vi "Binomial CDF.vi"(9 "p":dbl=0.02, 10 "n":i32=100, 11 "x":dbl) -> (0 "error":i32, 3 "cdf(x)":dbl=0.13261955589475294)   [LabVIEW 2020, in "NI_Gmath.lvlib"]
doc: "Computes the discrete cumulative distribution function (CDF), or the probability that the random variate X, where X describes the selected distribution type, takes on a value less than or equal to <B>x</B>. You must manually select the polymorphic instance to use."
uses:
  <vilib>/gmath/NI_Gmath.lvlib
  <vilib>/gmath/statdist.llb/st_error_code.ctl
  <vilib>/gmath/SpecialFunctions.llb/Incomplete Beta Function.vi
panel:
  # "Binomial CDF"
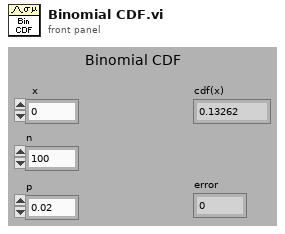
[diagram p1: front panel]
types:
  T1 = typedef "NI_Gmath.lvlib/st_error_code.ctl" = i32
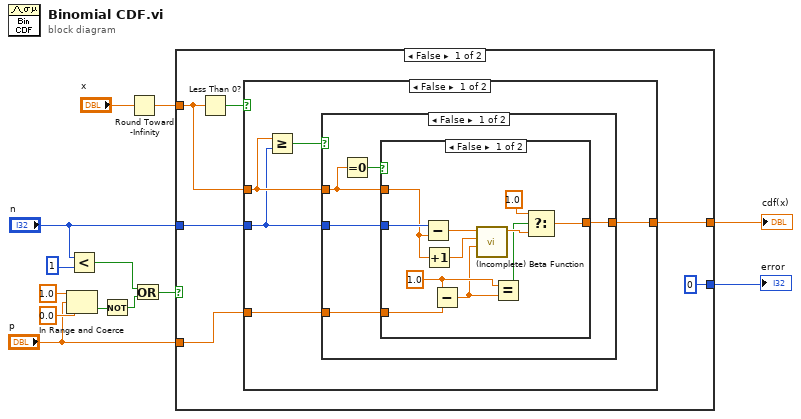
[diagram p0: block diagram]
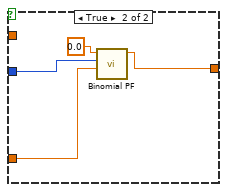
[diagram p2: hidden frame]
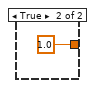
[diagram p3: hidden frame]
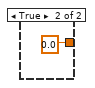
[diagram p4: hidden frame]
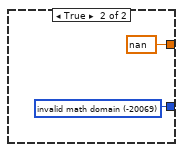
[diagram p5: hidden frame]
diagram:
  n1 = In Range and Coerce(upper limit=1.0, x="p", lower limit=0.0) -> (In Range?=w5:bool)  [unwired: 1 out]
  n2 = Less?(x="n", y=1) -> (x < y?=w3:bool)
  n3 = Not(x=w5) -> (.not. x?=w4:bool)
  n4 = Round Toward -Infinity(1:"x") -> (0:w1:dbl)
  n5 = Or(x=w3, y=w4) -> (x .or. y?=w8:bool)
  n6 = case shown="False" w8 {
    tunnel: [0 ("invalid math domain") w47] -> w13
    tunnel: [w18 nan] -> w12
    tunnel: w1 -> [w14 _]
    tunnel: "n" -> [w17 _]
    tunnel: "p" -> [w16 _]
    frame False {
      n7 = Less Than 0?(x=w14) -> (x < 0?=w15:bool)
      n8 = case shown="False" w15 {
        tunnel: [w23 0.0] -> w18
        tunnel: w14 -> [w22 _]
        tunnel: w17 -> [w21 _]
        tunnel: w16 -> [w20 _]
        frame False {
          n9 = Greater Or Equal?(x=w22, y=w21) -> (x >= y?=w24:bool)
          n10 = case shown="False" w24 {
            tunnel: [w26 1.0] -> w23
            tunnel: w22 -> [w25 _]
            tunnel: w21 -> [w28 _]
            tunnel: w20 -> [w27 _]
            frame False {
              n11 = Equal To 0?(x=w25) -> (x = 0?=w29:bool)
              n12 = case shown="False" w29 {
                tunnel: w28 -> [w40 w42]
                tunnel: w27 -> [w36 w43]
                tunnel: [w31 w41] -> w26
                tunnel: w25 -> [w38 _]
                frame False {
                  w35 = 1.0
                  n13 = Subtract(x=w40, y=w38) -> (x-y=w39:dbl)
                  n14 = Increment(x=w38) -> (x+1=w37:dbl)
                  n15 = Subtract(x=w35, y=w36) -> (x-y=w30:dbl)
                  n16 = call-poly <vilib>:"(Incomplete) Beta Function.vi"("a"=w30, "y"=w37, "x"=w39) -> ("b(x, y, a)"=w33:dbl)  [unwired: 8 in]
                  n17 = Equal?(x=w35, y=w30) -> (x = y?=w32:bool)
                  n18 = Select(t=1.0, s=w32, f=w33) -> (s? t:f=w31:dbl)
                }
                frame True {
                  n19 = call <vilib>:"Binomial PF.vi"("p"=w43, "n"=w42, "x"=0.0 ("a")) -> ("prob(x)"=w41:dbl)  [unwired: 7 in, 1 out]
                }
              }
            }
            frame True {
            }
          }
        }
        frame True {
        }
      }
    }
    frame True {
      w47 = T1 -20069 items=["invalid math domain"=-20069, "Fourier interpolation size m >= n"=-20070, "empty array"=-20003] ("stat interp error code")
    }
  }
  "cdf(x)" <- w12
  "error" <- w13
